vi "ReadHTTPHeader.vi"(8 "error in (no error)":errorcluster, 10 "timeout ms (25000)":i32=25000, 11 "WebSocket Connection in":refnum<k5>) -> (0 "error out":errorcluster, 2 "HTTP Header":string, 3 "WebSocket Connection out":refnum<k5>)   [LabVIEW 2014, in "QwaveSys RPi Training Library.lvlib" / "WebSockets.lvlib"]
doc: "WebSockets API 1.3.0.13\nSam Sharp - Intelligent Energy\nCopyright (c) 2015, Intelligent Energy"
uses:
  <vilib>/Q-Wave Systems/QwaveSys RPi Training Package (Demo)/Addons/WebSockets API/WebSockets/WebSockets.lvlib
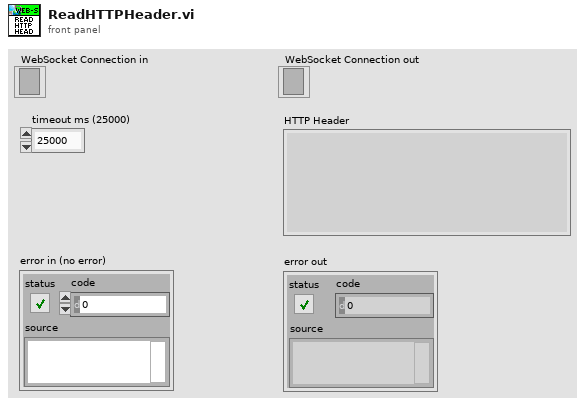
[diagram p1: front panel]
types:
  T1 = enum16{"Standard", "Buffered", "CRLF", "Immediate"}
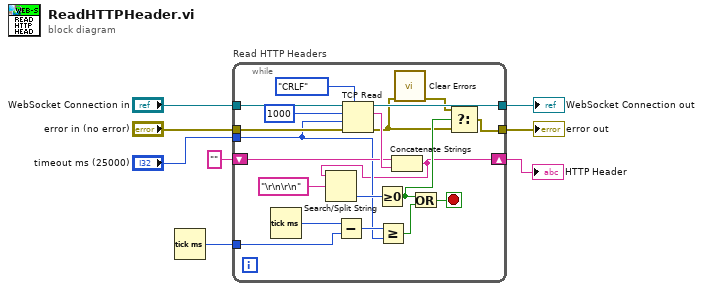
[diagram p0: block diagram]
diagram:
  n1 = Tick Count (ms)() -> (millisecond timer value=w8:u32)
  n2 = while "Read HTTP Headers" {
    tunnel: "WebSocket Connection in" -> [w28]
    tunnel: [w27] -> w2
    shift-right: [w9] -> w1
    shift-left: "" -> [w23]
    tunnel: "timeout ms (25000)" -> [w16]
    tunnel: [w10] -> w6
    tunnel: "error in (no error)" -> [w24]
    tunnel: w8 -> [w17]
    stop <- w22 stop-if-true
    n3 = Tick Count (ms)() -> (millisecond timer value=w18:u32)
    n4 = Subtract(x=w18, y=w17) -> (x-y=w20:u32)
    n5 = TCP Read(connection ID=w28, bytes to read=1000, error in (no error)=w24, 7:T1."CRLF" ("mode (standard)"), 9:w16) -> (connection ID out=w27:refnum<k5>, data out=w25:string, error out=w12:errorcluster)
    n6 = Greater Or Equal?(x=w20, y=w16) -> (x >= y?=w19:bool)
    n7 = Concatenate Strings(w23, w25) -> (w9:string)
    n8 = Search/Split String(string=w9, search string/char (-)="\r\n\r\n") -> (offset of match=w21:i32)  [unwired: 1 in, 2 out]
    n9 = Greater Or Equal To 0?(x=w21) -> (x >= 0?=w13:bool)
    n10 = call <vilib>:"Clear Errors.vi"("error in (no error)"=w12) -> ("error out"=w11:errorcluster)  [unwired: 5 in, 1 out]
    n11 = Or(x=w13, y=w19) -> (x .or. y?=w22:bool)
    n12 = Select(t=w11, s=w13, f=w12) -> (s? t:f=w10:errorcluster)
  }
  "error out" <- w6
  "WebSocket Connection out" <- w2
  "HTTP Header" <- w1
